vi "Sign_Setup.vi"(8 "error in (no error)":errorcluster, 11 "IB_MSI in":refnum<class "IB_MSI.lvclass">) -> (0 "error out":errorcluster, 3 "IB_MSI out":refnum<class "IB_MSI.lvclass">)   [LabVIEW 2020, in "IB_MSI.lvclass"]
uses:
  <vilib>/AppBuilder/IB_Classes/MSI/IB_MSI.lvclass
  <vilib>/AppBuilder/IB_Classes/MSI/IB_MSI.lvclass/IB_MSI.ctl
  <vilib>/AppBuilder/CodeSignAPI/CodeSignAPI.lvlib
  <vilib>/AppBuilder/IB_Classes/Installer/Installer.lvclass
  e:/builds/penguin/labview/branches/2020/dev/dist/vi.lib/AppBuilder/IB_Classes/Installer/Installer.lvclass
  e:/builds/penguin/labview/branches/2020/dev/dist/vi.lib/AppBuilder/IB_Classes/MSI/IB_MSI.lvclass
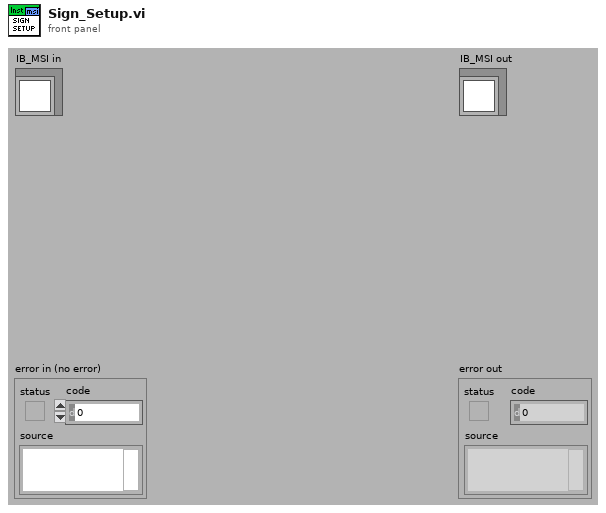
[diagram p1: front panel]
types:
  T1 = typedef "IB_Installer.ctl" = cluster{"Destination":refnum<class "IB_Destination.lvclass">[], "Source":refnum<class "IB_Source.lvclass">[], "buildObject":T2, "defaultDir":string, "platform":string, "author":string, "productName":string, "buildSpecName":string, "hide":bool, "requireLVDevSys":bool, "autoIncrement":bool, "includeError":bool, "readmeID":string, "buildLocation":path, "readmePath":path, "mediaSize":u16, "language":T3, "productVersion":T4, "preview":bool, "programmatic":bool, "progressBarEvents":T5, "userLog_Path":path, "shortcutAddresses":T7[], "EXE_Install Address":string, "EXE_Uninstall Address":string, "additional NIPaths":refnum<class "Dest_NI_NIPath.lvclass">[], "web service itemIDs":string[], "installerName":string}
  T2 = typedef "ItemRef.ctl" = u64
  T3 = typedef "CDK_sTypeDef_Languages.ctl" = u16
  T4 = typedef "CDK_sTypeDef_ProductVersion.ctl" = cluster{"Major":u8, "Minor":u8, "Update":u16}
  T5 = typedef "provcom_ProgressBar_Events.ctl" = cluster{"newJob":refnum<user-event>, "newItem":refnum<user-event>, "errorMsg":T6, "cancel":refnum<user-event>}
  T6 = typedef "mxLvBuildError.ctl" = refnum<user-event>
  T7 = typedef "CDK_sTypeDef_ShortcutAddress.ctl" = cluster{"file":string, "shortcut":string}
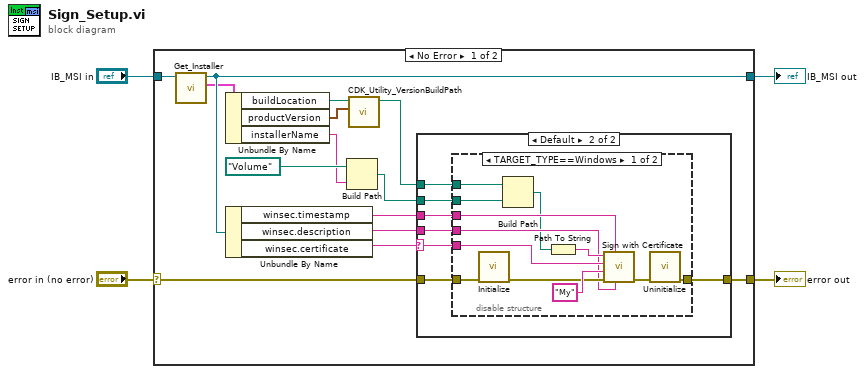
[diagram p0: block diagram]
diagram:
  n1 = case shown="No Error" "error in (no error)" {
    selector: "error in (no error)" -> [w15 w41]
    tunnel: [w14 w41] -> w3
    tunnel: [w12 w40] -> w1
    tunnel: "IB_MSI in" -> [w13 w40]
    frame No Error {
      n2 = call <vilib>:"Get_Installer.vi"("Installer in"=w13) -> ("data"=w11:T1, "Installer out"=w12:refnum<class "IB_MSI.lvclass">)  [unwired: 1 in, 8 out]
      n3 = Unbundle By Name(w11) -> ("buildLocation"=w7:path, "productVersion"=w6:T4, "installerName"=w8:string)
      n4 = Unbundle By Name(w12) -> ("winsec.timestamp"=w18:string, "winsec.description"=w17:string, "winsec.certificate"=w16:string)
      n5 = Build Path(base path=path "Volume", name or relative path=w8) -> (appended path=w10:path)
      n6 = call <resource>:"CDK_Utility_VersionBuildPath.vi"("ProductVersionIn"=w6, "build path in"=w7) -> ("build path out"=w5:path)  [unwired: 7 in, 2 out]
      n7 = case shown="Default" w16 {
        selector: w16 -> [_ w20]
        tunnel: w18 -> [_ w26]
        tunnel: w15 -> [w19 w25]
        tunnel: [w19 w24] -> w14
        tunnel: w17 -> [_ w23]
        tunnel: w5 -> [_ w22]
        tunnel: w10 -> [_ w21]
        frame "" {
          # "Do not sign if certificate is empty"
        }
        frame Default {
          n8 = disable-structure shown="TARGET_TYPE==Windows" {
            disable-tunnel: w26 -> [w34 _]
            disable-tunnel: w25 -> [w33 w39]
            disable-tunnel: [w32 w39] -> w24
            disable-tunnel: w20 -> [w31 _]
            disable-tunnel: w23 -> [w30 _]
            disable-tunnel: w22 -> [w29 _]
            disable-tunnel: w21 -> [w27 _]
            frame condition #0 (active) {
              n9 = call <vilib>:"Initialize.vi"("error in (no error)"=w33) -> ("error out"=w35:errorcluster)  [unwired: 10 out]
              n10 = Build Path(base path=w29, name or relative path=w27) -> (appended path=w28:path)
              n11 = Path To String(path=w28) -> (string=w37:string)
              n12 = call <vilib>:"Sign with Certificate.vi"("url"=w30, "tsa"=w34, "error in (no error)"=w35, "store"="My", "certname"=w31, "filepath"=w37) -> ("error out"=w36:errorcluster)  [unwired: 5 out]
              n13 = call <vilib>:"Uninitialize.vi"("error in (no error)"=w36) -> ("error out"=w32:errorcluster)  [unwired: 10 out]
            }
            frame condition #1 {
            }
          }
        }
      }
    }
    frame Error {
    }
  }
  "error out" <- w3
  "IB_MSI out" <- w1
